vi "Keithley Sweep and Acquire Measurements.vi"(4 "Source Delay (s)":dbl=0.1, 5 "Sweep Direction":u16(ring) items=["Low to high", "High to low"], 6 "Number of Points":u32=5, 7 "Maximum Amplitude":dbl=2.0, 8 "Minimum Amplitude":dbl=1.0, 9 "VISA resource name":refnum<visa-resource-name>) -> (0 "Measurement Complete":bool, 2 "Data Array":dbl[][](array[numeric]), 3 "VISA resource name out":refnum<visa-resource-name>)   [LabVIEW 2011]
doc: "Configures a sweep and takes voltage and current readings at each point."
uses:
  C:/Program Files (x86)/National Instruments/LabVIEW 2009/instr.lib/Keithley 24XX/Public/Data/Read (Multiple Points).vi
  C:/Program Files (x86)/National Instruments/LabVIEW 2009/instr.lib/Keithley 24XX/Keithley 24XX.lvlib
panel:
  in  "Source Mode  (0: Voltage)":u16(ring) items=["Voltage", "Current"]
  in  "Timeout (10000 ms)":i32=10000 format="%#.6g"
  in  "Compliance  Level":dbl=0.1
  # "(c) 2006 National Instruments.  ALL RIGHTS RESERVED."
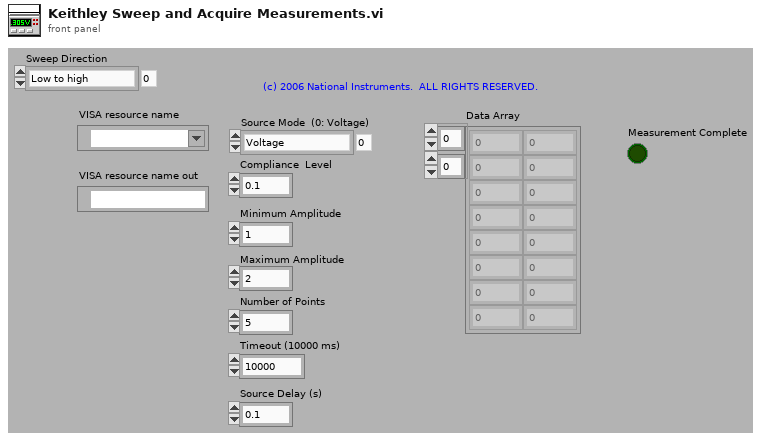
[diagram p1: front panel]
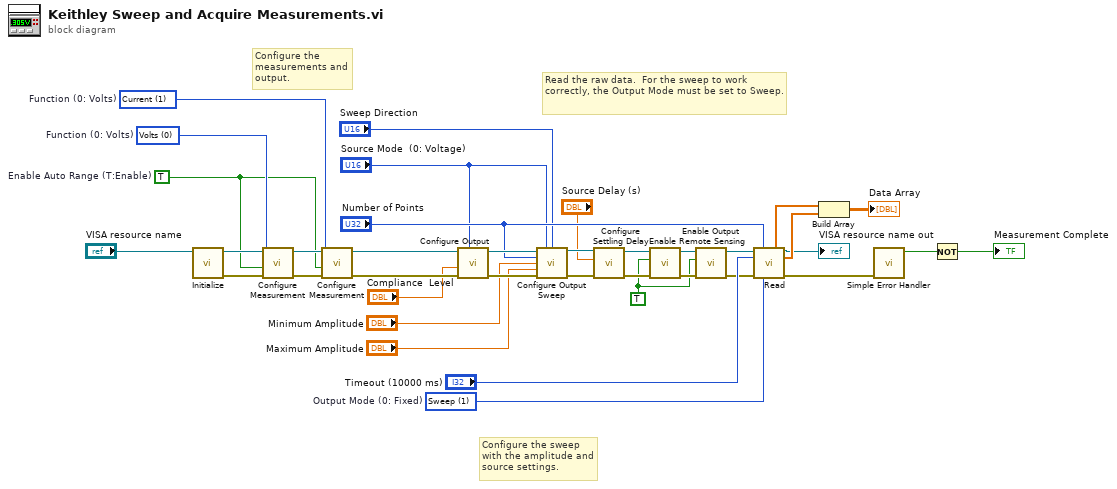
[diagram p0: block diagram]
diagram:
  w1 = TRUE ("Enable Output (T: Enable)")
  w16 = TRUE  # Enable Auto Range (T:Enable)
  w17 = u16 1 items=["Volts", "Current", "Resistance"]  # Function (0: Volts)
  w18 = u16 0 items=["Volts", "Current", "Resistance"]  # Function (0: Volts)
  w22 = u16 1 items=["Fixed", "Sweep", "List"]  # Output Mode (0: Fixed)
  # "Read the raw data.  For the sweep to work correctly, the Output Mode must be set to Sweep."
  # "Configure the sweep with the amplitude and source settings."
  # "Configure the measurements and output."
  n1 = call "Initialize.vi"("VISA resource name"="VISA resource name") -> ("error out"=w36:errorcluster, "VISA resource name out"=w37:refnum<visa-resource-name>)  [unwired: 9 in]
  n2 = call "Configure Measurement.vi"("error in (no error)"=w36, "Enable Auto Range (T:Enable)"=w16, "Function (0: Volts)"=w18, "VISA resource name"=w37) -> ("error out"=w35:errorcluster, "VISA resource name out"=w34:refnum<visa-resource-name>)  [unwired: 6 in]
  n3 = call "Configure Measurement.vi"("error in (no error)"=w35, "Enable Auto Range (T:Enable)"=w16, "Function (0: Volts)"=w17, "VISA resource name"=w34) -> ("error out"=w32:errorcluster, "VISA resource name out"=w33:refnum<visa-resource-name>)  [unwired: 6 in]
  n4 = call "Configure Output.vi"("Source Mode  (0: Voltage)"="Source Mode  (0: Voltage)", "error in (no error)"=w32, "Compliance  Level (0.1)"="Compliance  Level", "VISA resource name"=w33) -> ("error out"=w31:errorcluster, "VISA resource name out"=w30:refnum<visa-resource-name>)  [unwired: 6 in]
  n5 = call "Configure Output Sweep.vi"("VISA resource name"=w30, "Source Mode  (0: Voltage)"="Source Mode  (0: Voltage)", "Sweep Direction  (0: Ascending)"="Sweep Direction", "Number of Points (5)"="Number of Points", "Minimum Amplitude (1)"="Minimum Amplitude", "Maximum Amplitude (2)"="Maximum Amplitude", "error in (no error)"=w31) -> ("VISA resource name out"=w8:refnum<visa-resource-name>, "error out"=w7:errorcluster)  [unwired: 7 in]
  n6 = call "Configure Settling Delay.vi"("error in (no error)"=w7, "Manual Settling Delay (0 sec)"="Source Delay (s)", "VISA resource name"=w8) -> ("error out"=w4:errorcluster, "VISA resource name out"=w5:refnum<visa-resource-name>)  [unwired: 7 in]
  n7 = call <instrlib>:"Enable Remote Sensing.vi"("error in (no error)"=w4, "Enable Remote Sensing (T: Enable)"=w1, "VISA resource name"=w5) -> ("error out"=w2:errorcluster, "VISA resource name out"=w3:refnum<visa-resource-name>)  [unwired: 7 in]
  n8 = call "Enable Output.vi"("error in (no error)"=w2, "Enable Output (T: Enable)"=w1, "VISA resource name"=w3) -> ("error out"=w21:errorcluster, "VISA resource name out"=w20:refnum<visa-resource-name>)  [unwired: 7 in]
  n9 = call-poly "Read.vi"("VISA resource name"=w20, "Sample Count (1)"="Number of Points", "Timeout (10000 ms)"="Timeout (10000 ms)", "error in (no error)"=w21, "Output Mode (0: Fixed)"=w22) -> ("Voltage"=w26:sgl[], "VISA resource name out"=→"VISA resource name out":refnum<visa-resource-name>, "Current"=w25:sgl[], "error out"=w13:errorcluster)  [unwired: 4 in, 3 out]
  n10 = Build Array(w26, w25) -> (→"Data Array":sgl[][])
  n11 = call <vilib>:"Simple Error Handler.vi"("error in (no error)"=w13) -> ("error?"=w11:bool)  [unwired: 4 in, 4 out]
  n12 = Not(x=w11) -> (.not. x?=→"Measurement Complete":bool)
